vi "Color_GreenQuotes.vi"(11 "String in":refnum<vi>) -> (3 "String out":refnum<vi>)   [LabVIEW 2021]
uses:
  Color_Globals.vi
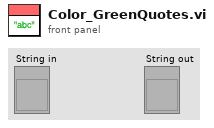
[diagram p1: front panel]
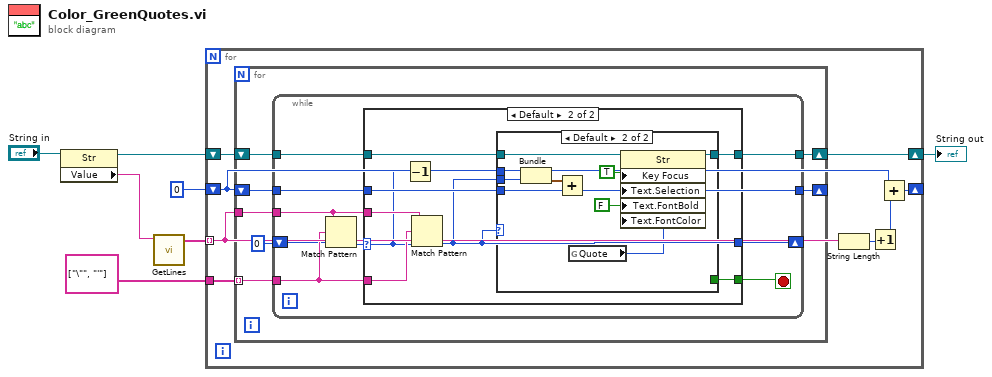
[diagram p0: block diagram]
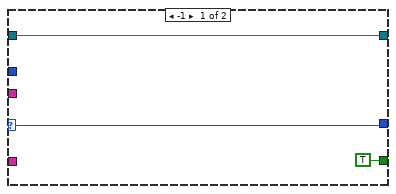
[diagram p2: hidden frame]
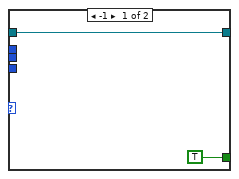
[diagram p3: hidden frame]
diagram:
  n1 = property on="Property Node" class="Str"(reference="String in") -> (reference out=w4:refnum<vi>, "Value"=w2:string)  [unwired: 1 in, 1 out]
  n2 = call "GetLines.vi"("String"=w2) -> ("Array"=w1:string[])  [unwired: 10 in]
  n3 = for {
    tunnel: string[] ["\"", "'"] -> [w14]
    shift-right: [w13] -> w3
    shift-left: w4 -> [w15]
    tunnel: w1 -> [w8] mode=indexing
    shift-right: [w11] -> _
    shift-left: 0 -> [w10]
    n4 = for {
      tunnel: w8 -> [w19]
      tunnel: w14 -> [w20] mode=indexing
      shift-right: [w21] -> w13
      shift-left: w15 -> [w22]
      shift-right: [w17] -> _
      shift-left: w10 -> [w18]
      n5 = while {
        tunnel: w19 -> [w29]
        shift-right: [w31] -> _
        shift-left: 0 -> [w23]
        tunnel: w22 -> [w30]
        tunnel: [w28] -> w21
        tunnel: w20 -> [w26]
        tunnel: w18 -> [w24]
        tunnel: [w24] -> w17
        stop <- w27 stop-if-true
        n6 = Match Pattern(string=w29, regular expression=w26, offset (0)=w23) -> (offset past match=w25:i32)  [unwired: 3 out]
        n7 = case shown="Default" w25 {
          selector: w25 -> [w33 w37]
          tunnel: [w33 w40] -> w31
          tunnel: w30 -> [w34 w43]
          tunnel: w29 -> [_ w42]
          tunnel: [w34 w41] -> w28
          tunnel: [TRUE w39] -> w27
          tunnel: w26 -> [_ w38]
          tunnel: w24 -> [_ w36]
          frame -1 {
          }
          frame Default {
            n8 = Decrement(x=w37) -> (x-1=w35:i32)
            n9 = Match Pattern(string=w42, regular expression=w38, offset (0)=w37) -> (offset past match=w40:i32)  [unwired: 3 out]
            n10 = case shown="Default" w40 {
              tunnel: w40 -> [_ w55]
              tunnel: w43 -> [w44 w52]
              tunnel: [w44 w51] -> w41
              tunnel: [TRUE _] -> w39
              tunnel: w35 -> [_ w50]
              tunnel: w36 -> [_ w47]
              frame -1 {
              }
              frame Default {
                n11 = Bundle(w50, "offset past match"=w55) -> (w49:cluster{i32, "offset past match":i32})  [unwired: 1 in]
                n12 = Add(x=w49, y=w47) -> (x+y=w48:cluster{i32, "offset past match":i32})
                n13 = global read "Color_Globals.vi" "Quote"() -> (w46:u32)
                n14 = property on="Property Node" class="Str"(reference=w52, "Key Focus"=TRUE, "Text.Selection"=w48, "Text.FontBold"=FALSE ("Text.Font:Bold"), "Text.FontColor"=w46) -> (reference out=w51:refnum<vi>)  [unwired: 1 in, 1 out]
              }
            }
          }
        }
      }
    }
    n15 = String Length(string=w8) -> (length=w12:i32)
    n16 = Increment(x=w12) -> (x+1=w9:i32)
    n17 = Add(x=w10, y=w9) -> (x+y=w11:i32)
  }
  "String out" <- w3
